vi "mediaIntesecaoCamerasYellows.vi"(11 "Array":T4[](array[typedef]) {"robots_blue"."height" format="%+4.3f"; "robots_blue"."pixel_y" format="%+4.3f"; "robots_blue"."pixel_x" format="%+4.3f"; "robots_blue"."orientation" format="%+4.3f"; "robots_blue"."y" format="%+4.3f"; "robots_blue"."confidence" format="%4.3f"; "robots_blue"."x" format="%+4.3f"; "robots_yellow"."height" format="%+4.3f"; "robots_yellow"."pixel_y" format="%+4.3f"; "robots_yellow"."pixel_x" format="%+4.3f"; "robots_yellow"."orientation" format="%+4.3f"; "robots_yellow"."y" format="%+4.3f"; "robots_yellow"."confidence" format="%4.3f"; "robots_yellow"."x" format="%+4.3f"}) -> (3 "Array 2":T1[](array[typedef]) {"height" format="%+4.3f"; "pixel_y" format="%+4.3f"; "pixel_x" format="%+4.3f"; "orientation" format="%+4.3f"; "y" format="%+4.3f"; "confidence" format="%4.3f"; "x" format="%+4.3f"})   [LabVIEW 2018]
uses:
  SSL Detection Frame.ctl
  SSL Detection Robot.ctl
  <vilib>/Analysis/Matrix/Datatypes/RealMatrix.ctl
  SSL Detection Ball.ctl
  <vilib>/Analysis/Matrix/NI_Matrix.lvlib
panel:
  in  "Field Size 2":T3
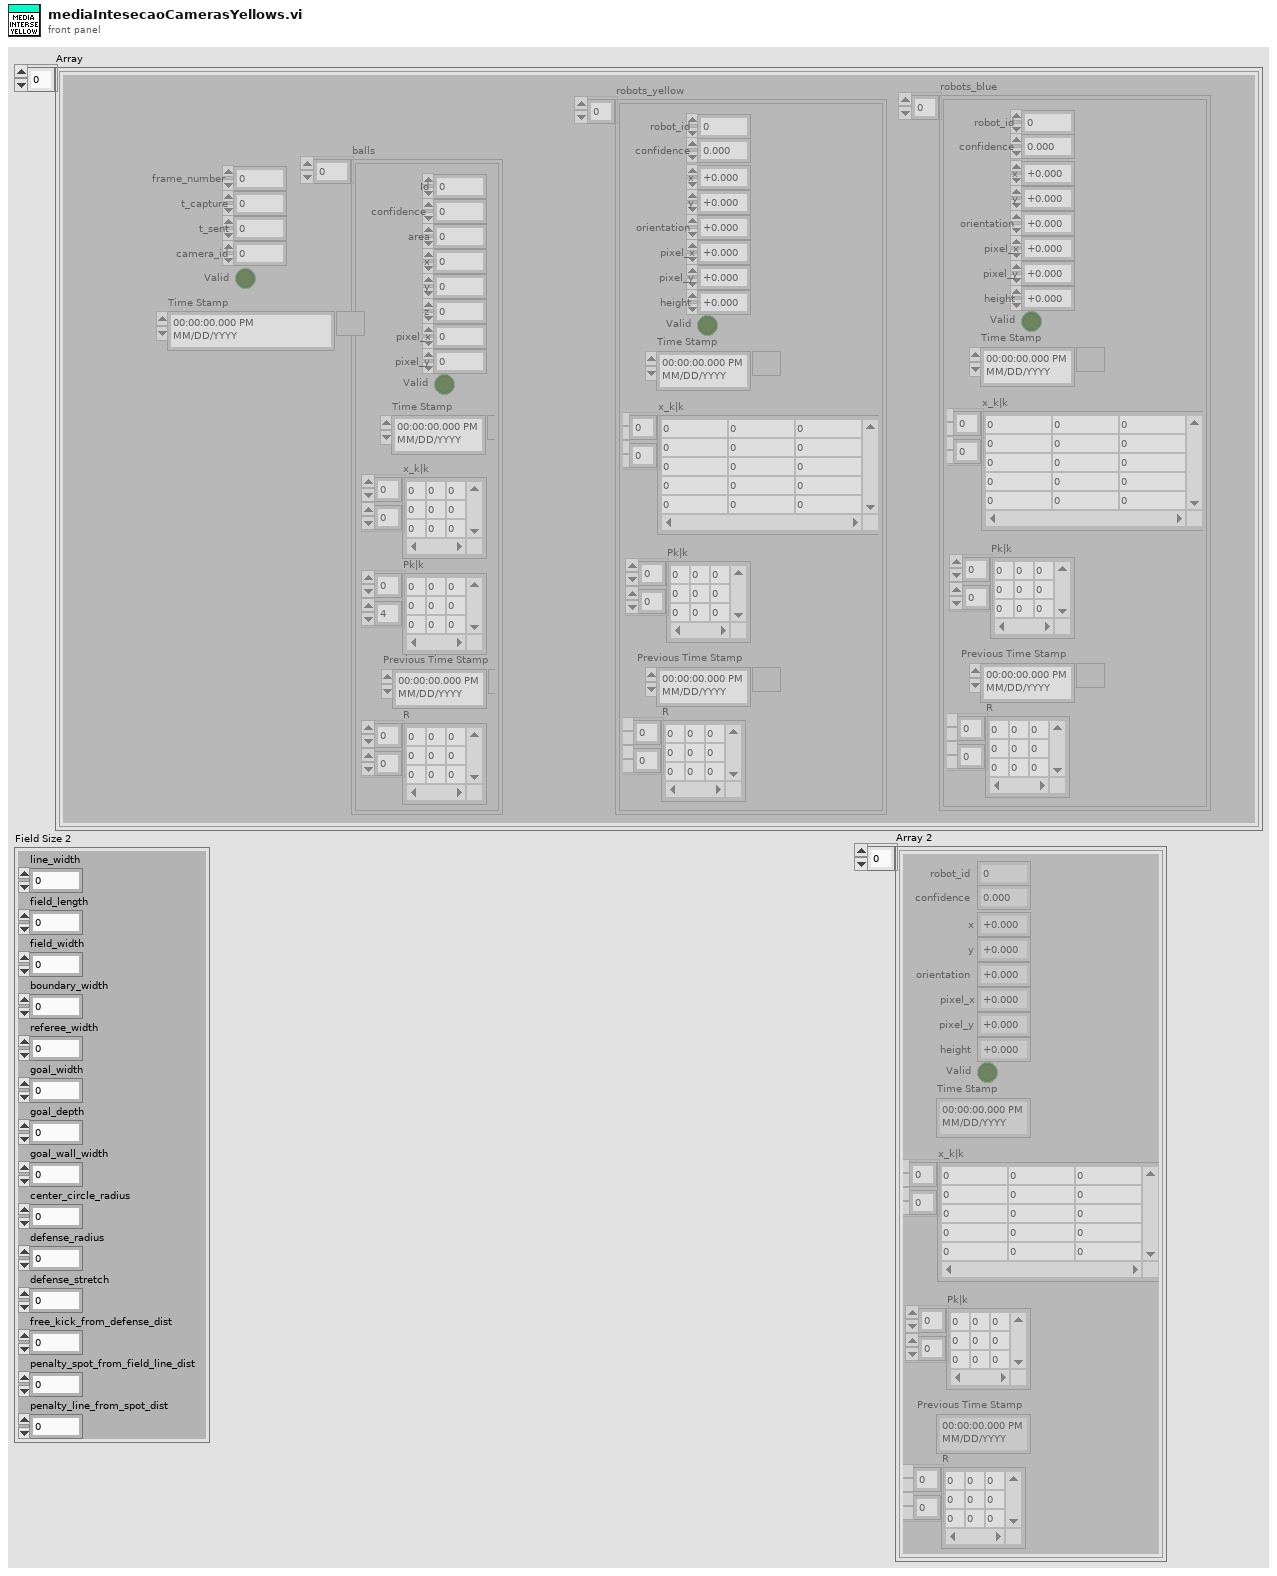
[diagram p1: front panel]
types:
  T1 = typedef "SSL Detection Robot.ctl" = cluster{"x":sgl, "robot_id":u32, "confidence":sgl, "y":sgl, "orientation":sgl, "pixel_x":sgl, "pixel_y":sgl, "height":sgl, "Valid":bool, "Time Stamp":timestamp, "x_k|k":T2, "Pk|k":T2, "Previous Time Stamp":timestamp, "R":T2}
  T2 = typedef "NI_Matrix.lvlib/RealMatrix.ctl" = dbl[][]
  T3 = cluster{"line_width":u32, "field_length":u32, "field_width":u32, "boundary_width":u32, "referee_width":u32, "goal_width":u32, "goal_depth":u32, "goal_wall_width":u32, "center_circle_radius":u32, "defense_radius":u32, "defense_stretch":u32, "free_kick_from_defense_dist":u32, "penalty_spot_from_field_line_dist":u32, "penalty_line_from_spot_dist":u32}
  T4 = typedef "SSL Detection Frame.ctl" = cluster{"frame_number":u32, "t_capture":dbl, "t_sent":dbl, "camera_id":u32, "robots_yellow":T1[], "robots_blue":T1[], "balls":T5[], "Valid":bool, "Time Stamp":timestamp}
  T5 = typedef "SSL Detection Ball.ctl" = cluster{"x":sgl, "area":u32, "confidence":sgl, "y":sgl, "z":sgl, "pixel_x":sgl, "pixel_y":sgl, "Valid":bool, "Time Stamp":timestamp, "x_k|k":T2, "Pk|k":T2, "Id":u32, "Previous Time Stamp":timestamp, "R":T2}
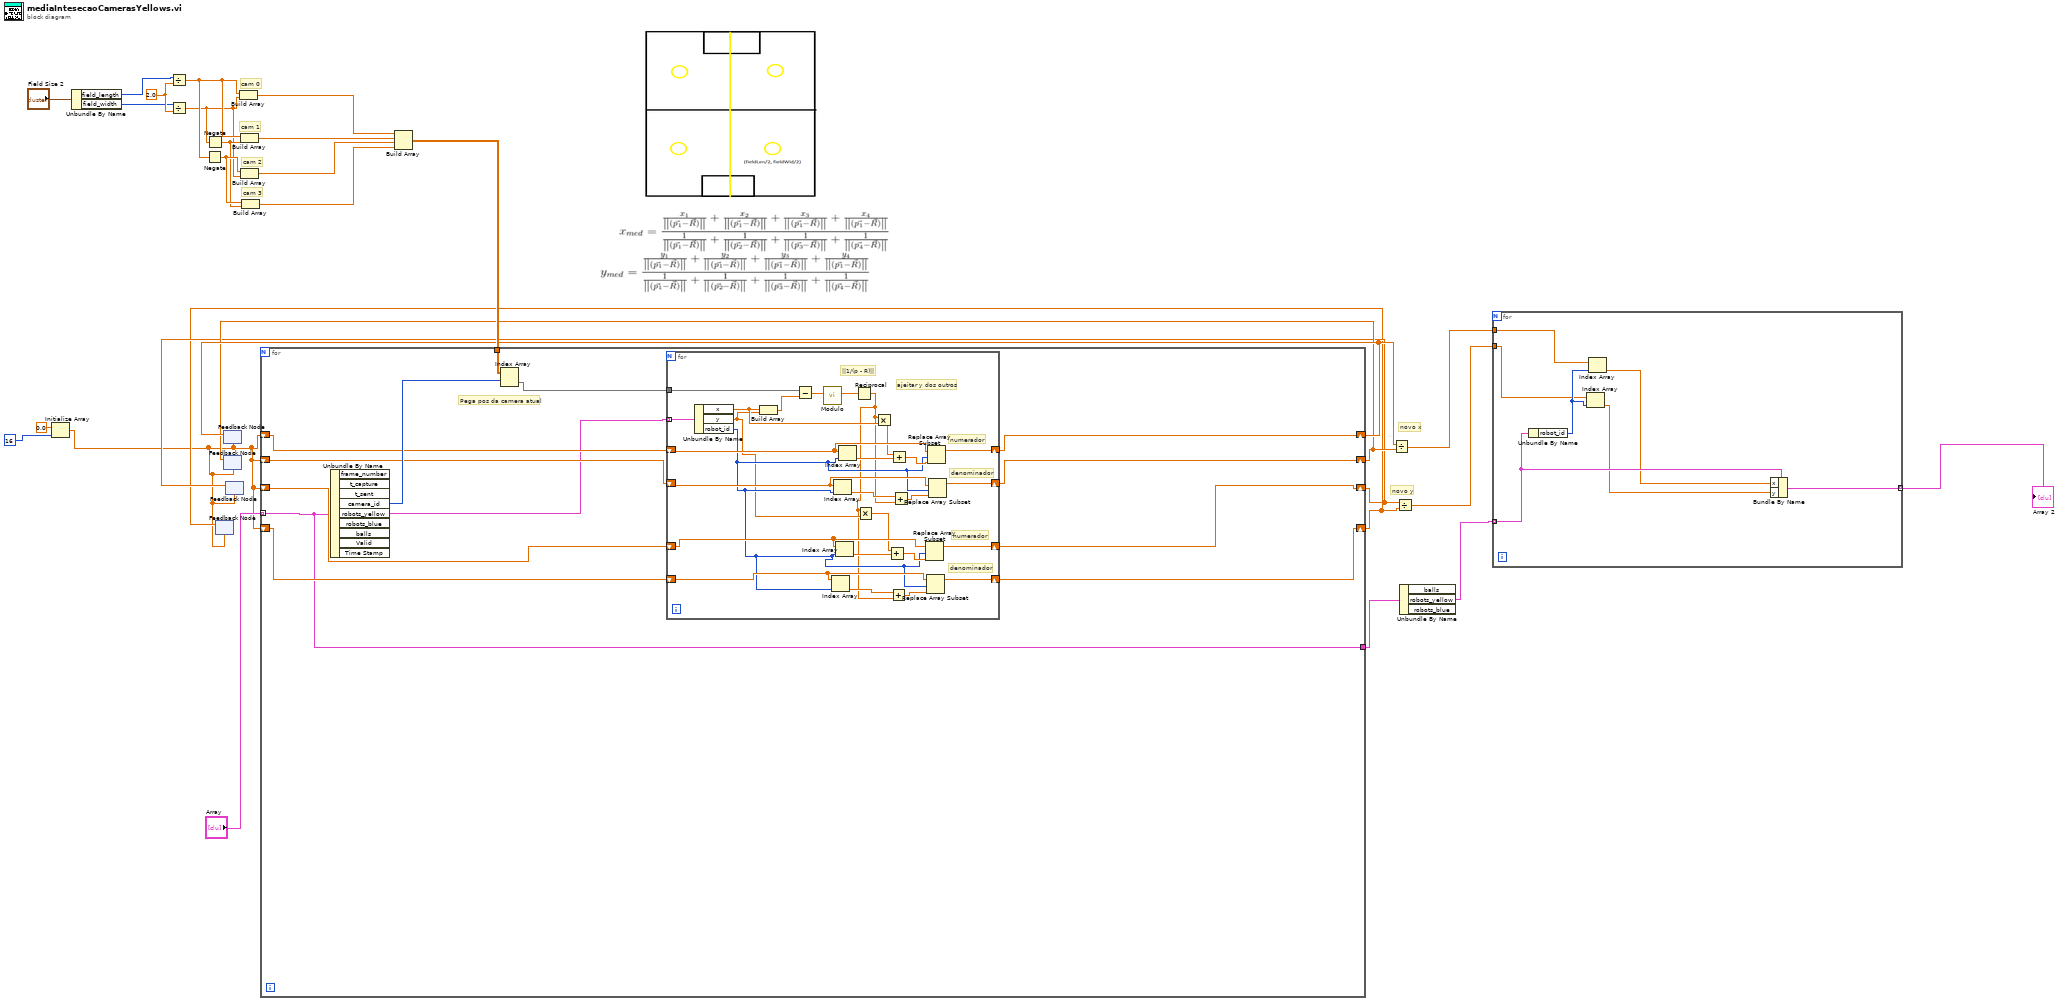
[diagram p0: block diagram]
diagram:
  w24 = 2.0 ("y")
  # "novo y"
  # "novo x"
  # "cam 3"
  # "cam 2"
  # "cam 1"
  # "cam 0"
  n1 = Initialize Array(0.0 ("element"), 16 ("dimension size")) -> (w1:dbl[])
  n2 = Unbundle By Name("Field Size 2") -> ("field_length"=w23:u32, "field_width"=w22:u32)
  n3 = Divide(x=w23, y=w24) -> (x/y=w20:dbl)
  n4 = Divide(x=w22, y=w24) -> (x/y=w18:dbl)
  n5 = Negate(x=w20) -> (-x=w21:dbl)
  n6 = Negate(x=w18) -> (-x=w19:dbl)
  n7 = feedback #1(w1) -> ()  [unwired: 1 in]
  n8 = feedback #2(w1) -> ()  [unwired: 1 in]
  n9 = feedback #3(w1) -> ()  [unwired: 1 in]
  n10 = feedback #4(w1) -> ()  [unwired: 1 in]
  n11 = Build Array(w20, w18) -> (w17:dbl[])
  n12 = Build Array(w20, w19) -> (w16:dbl[])
  n13 = Build Array(w21, w18) -> (w15:dbl[])
  n14 = Build Array(w21, w19) -> (w14:dbl[])
  n15 = Build Array(w17, w16, w15, w14) -> (w13:dbl[][])
  n16 = for {
    tunnel: "Array" -> [w27] mode=indexing
    tunnel: w13 -> [w39]
    shift-right: [w34] -> w5
    shift-left: w1 -> [w36]
    shift-right: [w33] -> w4
    shift-left: w1 -> [w35]
    shift-right: [w30] -> w3
    shift-left: w1 -> [w32]
    shift-right: [w29] -> w2
    shift-left: w1 -> [w31]
    tunnel: [w27] -> w6
    # "Pega pos da camera atual"
    n17 = Unbundle By Name(w27) -> ("camera_id"=w38:u32, "robots_yellow"=w28:T1[])  [unwired: 7 out]
    n18 = Index Array(array=w39, index (row)=w38) -> (element=w37:dbl[])  [unwired: 1 in]
    n19 = for {
      tunnel: w28 -> [w66] mode=indexing
      tunnel: w37 -> [w64]
      shift-right: [w60] -> w34
      shift-left: w36 -> [w58]
      shift-right: [w59] -> w33
      shift-left: w35 -> [w54]
      shift-right: [w44] -> w30
      shift-left: w32 -> [w47]
      shift-right: [w43] -> w29
      shift-left: w31 -> [w46]
      # "ajeitar y dos outros"
      # "denominador"
      # "numerador"
      # "denominador"
      # "numerador"
      # "||1/(p - R)||"
      n20 = Unbundle By Name(w66) -> ("x"=w61:sgl, "y"=w42:sgl, "robot_id"=w45:u32)
      n21 = Build Array(w61, w42) -> (w65:sgl[])
      n22 = Subtract(x=w64, y=w65) -> (x-y=w63:dbl[])
      n23 = call "Modulo.vi"("2D vector"=w63) -> ("Modulo"=w62:dbl)  [unwired: 10 in]
      n24 = Index Array(array=w46, index=w45) -> (element=w49:dbl)
      n25 = Index Array(array=w54, index=w45) -> (element=w53:dbl)
      n26 = Index Array(array=w47, index=w45) -> (element=w51:dbl)
      n27 = Index Array(array=w58, index=w45) -> (element=w56:dbl)
      n28 = Reciprocal(x=w62) -> (1/x=w40:dbl)
      n29 = Multiply(x=w40, y=w42) -> (x*y=w41:dbl)
      n30 = Multiply(x=w40, y=w61) -> (x*y=w57:dbl)
      n31 = Add(x=w41, y=w51) -> (x+y=w50:dbl)
      n32 = Add(x=w49, y=w40) -> (x+y=w48:dbl)
      n33 = Add(x=w57, y=w56) -> (x+y=w55:dbl)
      n34 = Add(x=w53, y=w40) -> (x+y=w52:dbl)
      n35 = Replace Array Subset(array=w47, new element=w50, index=w45) -> (w44:dbl[])
      n36 = Replace Array Subset(array=w46, new element=w48, index=w45) -> (w43:dbl[])
      n37 = Replace Array Subset(array=w58, new element=w55, index=w45) -> (w60:dbl[])
      n38 = Replace Array Subset(array=w54, new element=w52, index=w45) -> (w59:dbl[])
    }
  }
  n39 = feedback-in #1(w2) -> ()
  n40 = feedback-in #2(w5) -> ()
  n41 = feedback-in #3(w4) -> ()
  n42 = feedback-in #4(w3) -> ()
  n43 = Divide(x=w5, y=w4) -> (x/y=w10:dbl[])
  n44 = Divide(x=w3, y=w2) -> (x/y=w9:dbl[])
  n45 = Unbundle By Name(w6) -> ("robots_yellow"=w8:T1[])  [unwired: 2 out]
  n46 = for {
    tunnel: w10 -> [w72]
    tunnel: w9 -> [w70]
    tunnel: w8 -> [w73] mode=indexing
    tunnel: [w67] -> w7 mode=indexing
    n47 = Unbundle By Name(w73) -> ("robot_id"=w71:u32)
    n48 = Index Array(array=w70, index=w71) -> (element=w68:dbl)
    n49 = Index Array(array=w72, index=w71) -> (element=w69:dbl)
    n50 = Bundle By Name(cluster=w73, "x"=w69, "y"=w68) -> (w67:T1)
  }
  "Array 2" <- w7
